vi "uTransport_SendMsg Core.vi"(8 "error in (no error)":errorcluster, 10 "Msg":refnum<class "uMsg.lvclass">, 11 "uClient_Publisher in":refnum<class "uClient_Publisher.lvclass">) -> (0 "error out":errorcluster, 3 "uClient_Publisher out":refnum<class "uClient_Publisher.lvclass">)   [LabVIEW 2021, in "uFramework.lvlib" / "uClient_Publisher.lvclass"]
uses:
  uMsg/uMsg.lvclass
  uClient_Publisher.lvclass
  uClient_Publisher.lvclass/uClient_Publisher.ctl
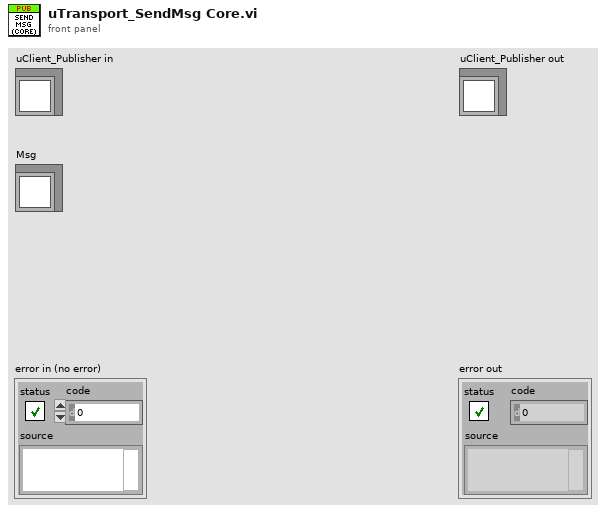
[diagram p1: front panel]
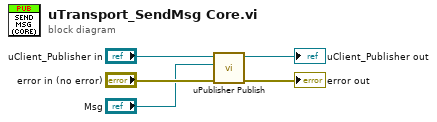
[diagram p0: block diagram]
diagram:
  n1 = call "uPublisher Publish.vi"("error in (no error)"="error in (no error)", "uMsg"="Msg", "uClient_Publisher in"="uClient_Publisher in") -> ("error out"=→"error out":errorcluster, "uClient_Publisher out"=→"uClient_Publisher out":refnum<class "uClient_Publisher.lvclass">)  [unwired: 7 in]
